vi "translatePolarityValues.vi"(0 "PMX4CXSAController in":refnum<class "PMX4CXSAController.lvclass">, 1 "simple_actions":T3, 2 "polarity_value (in)":u32, 3 "polarity_items (in)":T1[](array[typedef]), 5 "error in (no error)":errorcluster) -> (14 "PMX4CXSAController out":refnum<class "PMX4CXSAController.lvclass">, 16 "polarity_value (out)":u32, 17 "polarity_items (out)":T1[](array[typedef]), 19 "error out":errorcluster)   [LabVIEW 2020, in "classes.lvlib" / "PMX4CXSAController.lvclass"]
doc: "Produced By:\n\n<B>Kod Integrations, LLC</B>\n4835 Marianne Drive\nMount Airy, MD 21771\nhttp://www.kodintegrations.com\nemail: info@kodintegrations.com\nphone: (240) 687-1288"
uses:
  PMX4CXSAController.lvclass
  simple_actions.ctl
  polarity_item.ctl
  polarity.ctl
  common.lvlib
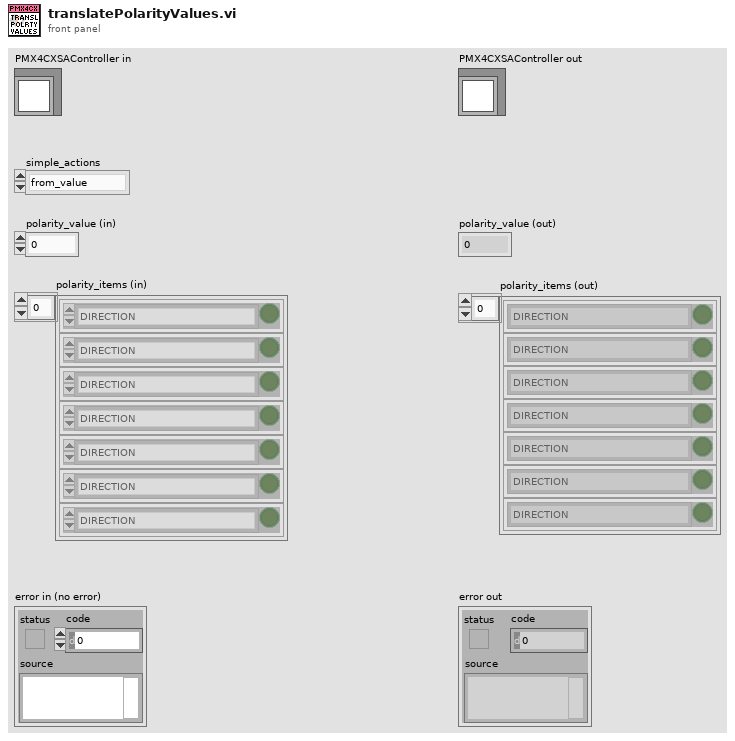
[diagram p1: front panel]
types:
  T1 = typedef "common.lvlib/polarity_item.ctl" = cluster{"item":T2, "status":bool}
  T2 = typedef "common.lvlib/polarity.ctl" = enum16{"DIRECTION", "LIMIT", "HOME", "DIG_OUT", "DIG_IN", "ENABLE_OUT", "JUMP_ERR", "LATCH", "Z-CHAN_INDEX", "ENCODER_DECODING:1X", "ENCODER_DECODING:2X", "ENCODER_DECODING:4X", "ALARM", "STANDALONE_ERR", "-", "<reserved/nc>"}
  T3 = typedef "common.lvlib/simple_actions.ctl" = enum16{"from_value", "to_value"}
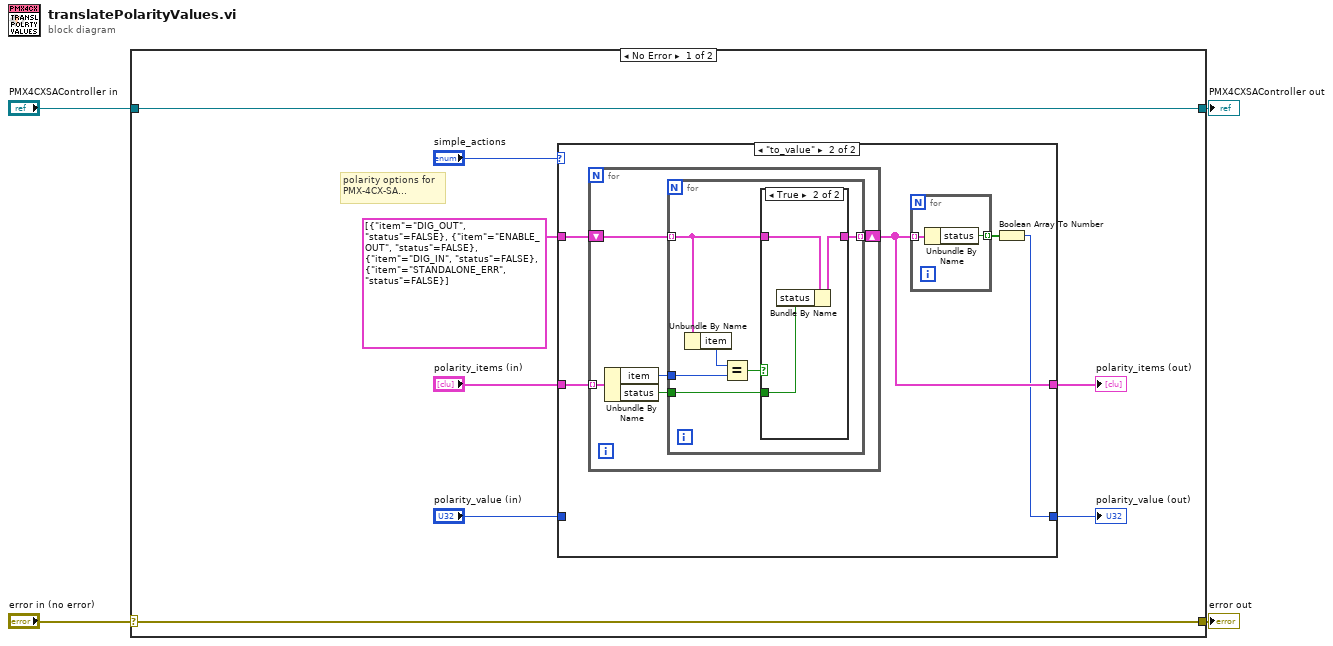
[diagram p0: block diagram]
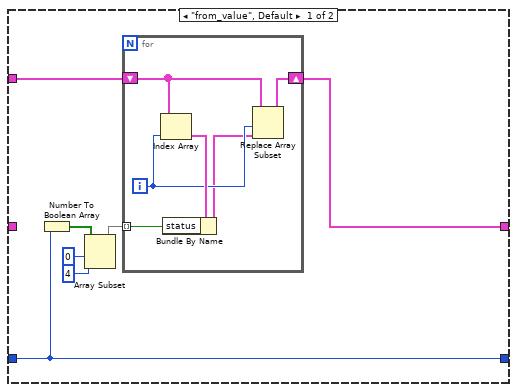
[diagram p2: hidden frame]
diagram:
  n1 = case shown="No Error" "error in (no error)" {
    selector: "error in (no error)" -> [w11 w49]
    tunnel: [w11 w49] -> w3
    tunnel: [w12 w48] -> w1
    tunnel: "PMX4CXSAController in" -> [w12 w48]
    frame No Error {
      # "polarity options for\nPMX-4CX-SA..."
      n2 = case shown="\"to_value\"" "simple_actions" {
        tunnel: [w15 w29] -> w6
        tunnel: T1[] [{"item"=enum."DIG_OUT", "status"=FALSE}, {"item"=enum."ENABLE_OUT", "status"=FALSE}, {"item"=enum."DIG_IN", "status"=FALSE}, {"item"=enum."STANDALONE_ERR", "status"=FALSE}] ("polarity_items (in)") -> [w14 w30]
        tunnel: [w13 w27] -> w5
        tunnel: "polarity_items (in)" -> [_ w26]
        tunnel: "polarity_value (in)" -> [w13 _]
        frame "from_value", Default {
          n3 = Number To Boolean Array(number=w13) -> (Boolean array=w19:bool[])
          n4 = Array Subset(array=w19, index=0, length=4) -> (w16:bool[])
          n5 = for {
            shift-right: [w20] -> w15
            shift-left: w14 -> [w23]
            tunnel: w16 -> [w24] mode=indexing
            i -> [w22]
            n6 = Index Array(array=w23, index=w22) -> (element=w25:T1)
            n7 = Bundle By Name(cluster=w25, "status"=w24) -> (w21:T1)
            n8 = Replace Array Subset(array=w23, new element=w21, index=w22) -> (w20:T1[])
          }
        }
        frame "to_value" {
          n9 = for {
            shift-right: [w34] -> w29
            shift-left: w30 -> [w37]
            tunnel: w26 -> [w33] mode=indexing
            n10 = Unbundle By Name(w33) -> ("item"=w36:T2, "status"=w35:bool)
            n11 = for {
              tunnel: w37 -> [w41] mode=indexing
              tunnel: w36 -> [w38]
              tunnel: w35 -> [w40]
              tunnel: [w39] -> w34 mode=indexing
              n12 = Unbundle By Name(w41) -> ("item"=w43:T2)
              n13 = Equal?(x=w43, y=w38) -> (x = y?=w42:bool)
              n14 = case shown="True" w42 {
                tunnel: w41 -> [w44 w47]
                tunnel: w40 -> [_ w45]
                tunnel: [w44 w46] -> w39
                frame False {
                }
                frame True {
                  n15 = Bundle By Name(cluster=w47, "status"=w45) -> (w46:T1)
                }
              }
            }
          }
          n16 = for {
            tunnel: w29 -> [w32] mode=indexing
            tunnel: [w31] -> w28 mode=indexing
            n17 = Unbundle By Name(w32) -> ("status"=w31:bool)
          }
          n18 = Boolean Array To Number(Boolean array=w28) -> (number=w27:u32)
        }
      }
      "polarity_items (out)" <- w6
      "polarity_value (out)" <- w5
    }
    frame Error {
    }
  }
  "error out" <- w3
  "PMX4CXSAController out" <- w1
